vi "Timer.vi"(8 "State":refnum<queue>, 9 "error in":errorcluster, 11 "TimeQueue":refnum<queue>) -> ()   [LabVIEW 2018]
doc: "Riceve attraverso la coda TimeQueue i comandi per attivare/disattivare il timer e inoltra attraverso la coda State gli stati aggiornati del controller."
uses:
  TimeCluster.ctl
  MessageCluster.ctl
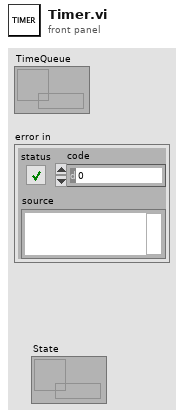
[diagram p1: front panel]
types:
  T1 = typedef "TimeCluster.ctl" = cluster{"run":bool, "destroy":bool, "Elapsed time":i32, "WaitTime":i32, "Ticktime":i32}
  T2 = typedef "MessageCluster.ctl" = cluster{"Message":string, "Temp":i32, "Stato":enum16{"On", "Off", "Preparation", "WaitTimer", "Ready"}}
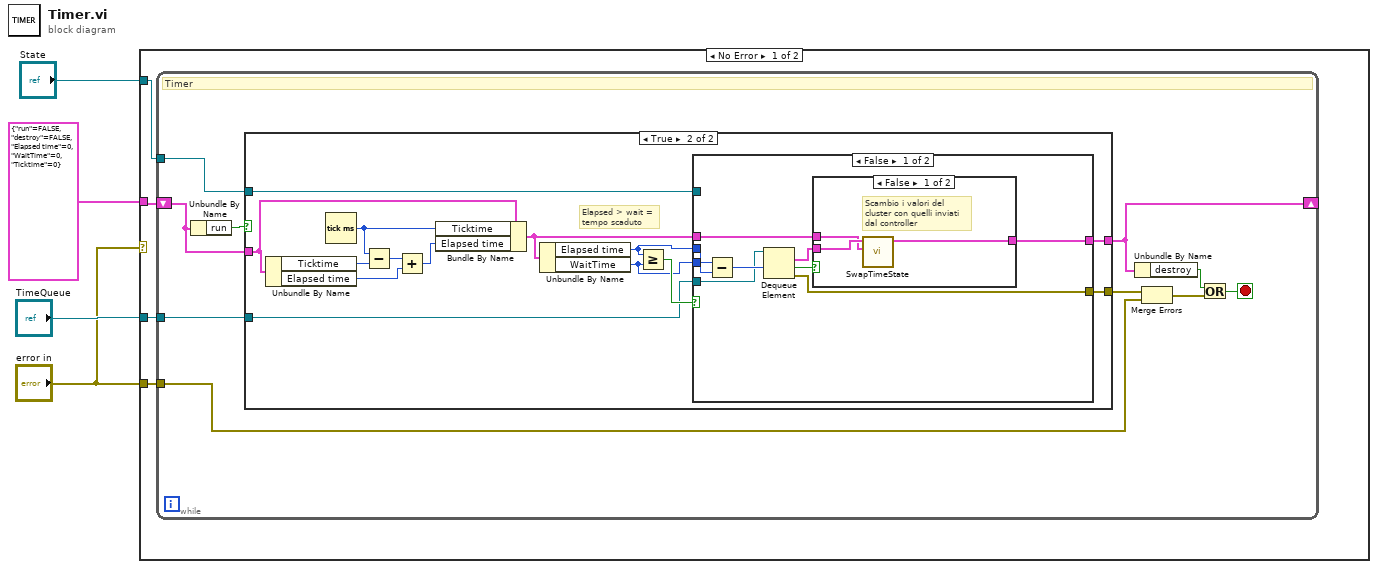
[diagram p0: block diagram]
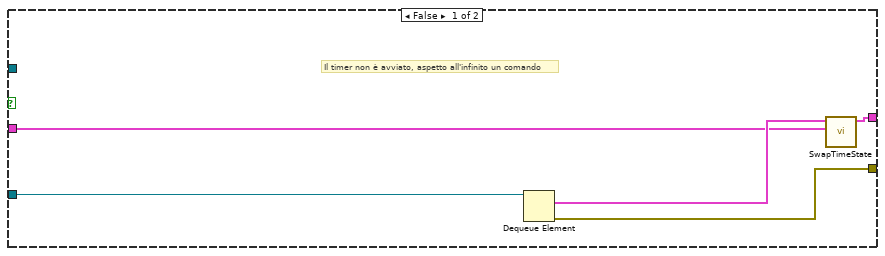
[diagram p2: hidden frame]
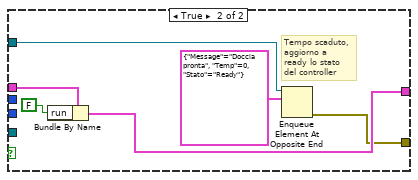
[diagram p4: hidden frame]
diagram:
  n1 = case shown="No Error" "error in" {
    tunnel: T1 {"run"=FALSE, "destroy"=FALSE, "Elapsed time"=0, "WaitTime"=0, "Ticktime"=0} -> [w8 _]
    tunnel: "TimeQueue" -> [w7 _]
    tunnel: "State" -> [w6 _]
    tunnel: "error in" -> [w5 _]
    frame No Error {
      n2 = while {
        shift-right: [w15] -> _
        shift-left: w8 -> [w17]
        tunnel: w7 -> [w16]
        tunnel: w6 -> [w14]
        tunnel: w5 -> [w9]
        stop <- w10 stop-if-true
        # "Timer"
        n3 = Unbundle By Name(w17) -> ("run"=w18:bool)
        n4 = case shown="True" w18 {
          tunnel: w17 -> [w21 w32]
          tunnel: w16 -> [w23 w28]
          tunnel: [w20 w26] -> w15
          tunnel: [w19 w25] -> w13
          tunnel: w14 -> [_ w24]
          frame False {
            # "Il timer non è avviato, aspetto all'infinito un comando"
            n5 = Dequeue Element(queue=w23) -> (element=w22:T1, error out=w19:errorcluster)  [unwired: 2 in, 2 out]
            n6 = call "SwapTimeState.vi"("Old cluster"=w21, "New cluster"=w22) -> ("Cluster out"=w20:T1)  [unwired: 9 in]
          }
          frame True {
            # "Elapsed > wait = \ntempo scaduto"
            n7 = Unbundle By Name(w32) -> ("Ticktime"=w37:i32, "Elapsed time"=w35:i32)
            n8 = Tick Count (ms)() -> (millisecond timer value=w33:u32)
            n9 = Subtract(x=w33, y=w37) -> (x-y=w36:u32)
            n10 = Add(x=w36, y=w35) -> (x+y=w34:u32)
            n11 = Bundle By Name(cluster=w32, "Ticktime"=w33, "Elapsed time"=w34) -> (w27:T1)
            n12 = Unbundle By Name(w27) -> ("Elapsed time"=w29:i32, "WaitTime"=w30:i32)
            n13 = Greater Or Equal?(x=w29, y=w30) -> (x >= y?=w31:bool)
            n14 = case shown="False" w31 {
              tunnel: w30 -> [w46 _]
              tunnel: w29 -> [w45 _]
              tunnel: w28 -> [w43 _]
              tunnel: w27 -> [w41 w54]
              tunnel: [w39 w53] -> w26
              tunnel: [w38 w51] -> w25
              tunnel: w24 -> [_ w52]
              frame False {
                n15 = Subtract(x=w46, y=w45) -> (x-y=w44:i32)
                n16 = Dequeue Element(queue=w43, timeout in ms (-1)=w44) -> (element=w40:T1, timed out?=w42:bool, error out=w38:errorcluster)  [unwired: 1 in, 1 out]
                n17 = case shown="False" w42 {
                  tunnel: w41 -> [w48 w50]
                  tunnel: w40 -> [w49 _]
                  tunnel: [w47 w50] -> w39
                  frame False {
                    # "Scambio i valori del \ncluster con quelli inviati\ndal controller"
                    n18 = call "SwapTimeState.vi"("Old cluster"=w48, "New cluster"=w49) -> ("Cluster out"=w47:T1)  [unwired: 9 in]
                  }
                  frame True {
                    # "Timeout scaduto, passo\nal prossimo giro"
                  }
                }
              }
              frame True {
                # "Tempo scaduto,\naggiorno a \nready lo stato\ndel controller"
                n19 = Bundle By Name(cluster=w54, "run"=FALSE) -> (w53:T1)
                n20 = Enqueue Element At Opposite End(queue=w52, element=T2 {"Message"="Doccia pronta", "Temp"=0, "Stato"=enum."Ready"} ("Message Cluster")) -> (error out=w51:errorcluster)  [unwired: 2 in, 2 out]
              }
            }
          }
        }
        n21 = Unbundle By Name(w15) -> ("destroy"=w11:bool)
        n22 = Merge Errors(w13, w9) -> (w12:errorcluster)
        n23 = Or(x=w11, y=w12) -> (x .or. y?=w10:bool)
      }
    }
    frame Error {
    }
  }
